vi "Treat Path for Platform.vi"(8 "error in (no error)":errorcluster, 11 "File Path":path) -> (0 "error out":errorcluster, 3 "Path for CLI":string)   [LabVIEW 2019, in "Command-Line Zip.lvlib"]
uses:
  Command-Line Zip.lvlib
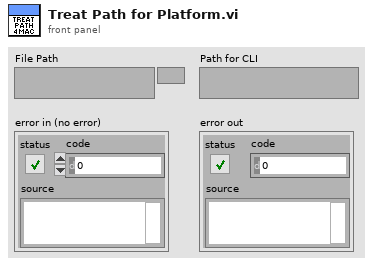
[diagram p1: front panel]
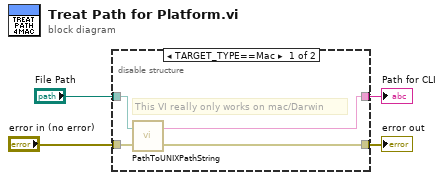
[diagram p0: block diagram]
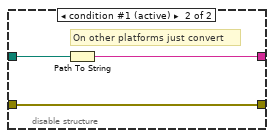
[diagram p2: hidden frame]
diagram:
  n1 = disable-structure shown="TARGET_TYPE==Mac" {
    disable-tunnel: [w8 w9] -> w1
    disable-tunnel: "error in (no error)" -> [w6 w9]
    disable-tunnel: "File Path" -> [w5 w11]
    disable-tunnel: [w7 w10] -> w4
    frame condition #0 {
      # "This VI really only works on mac/Darwin"
      n2 = call <vilib>:"PathToUNIXPathString.vi"("error in (no error)"=w6, "LV Path"=w5) -> ("error out"=w8:errorcluster, "UNIX Path"=w7:string)
    }
    frame condition #1 (active) {
      # "On other platforms just convert"
      n3 = Path To String(path=w11) -> (string=w10:string)
    }
  }
  "Path for CLI" <- w4
  "error out" <- w1
